vi "Initialize Hardware References.vi"(8 "error in (no error)":errorcluster, 11 "Hardware Resources in":T1={"VISA Refnum in"="", "Serial Configuration"={"Baud Rate"=460800, "Flow Control"=0}, "Voltage Level (0V)"=0.0} {"Serial Configuration"."Flow Control" items=["None", "XON/XOFF", "RTS/CTS", "XON/XOFF & RTS/CTS", "DTR/DSR", "XON/XOFF & DTR/DSR"]; "Serial Configuration"."Baud Rate" items=["9600"=9600, "19200"=19200, "38400"=38400, "57600"=57600, "115200"=115200, "230400"=230400, "460800"=460800]}) -> (0 "error out":errorcluster, 3 "Hardware Resources out":T1={"VISA Refnum in"="", "Serial Configuration"={"Baud Rate"=460800, "Flow Control"=0}, "Voltage Level (0V)"=0.0} {"Serial Configuration"."Flow Control" items=["None", "XON/XOFF", "RTS/CTS", "XON/XOFF & RTS/CTS", "DTR/DSR", "XON/XOFF & DTR/DSR"]; "Serial Configuration"."Baud Rate" items=["9600"=9600, "19200"=19200, "38400"=38400, "57600"=57600, "115200"=115200, "230400"=230400, "460800"=460800]})   [LabVIEW 2013, in "Cal Inst Acquisition.lvlib"]
doc: "Initialize the hardware references."
uses:
  Cal Inst Acquisition.lvlib
  Hardware Configuration.ctl
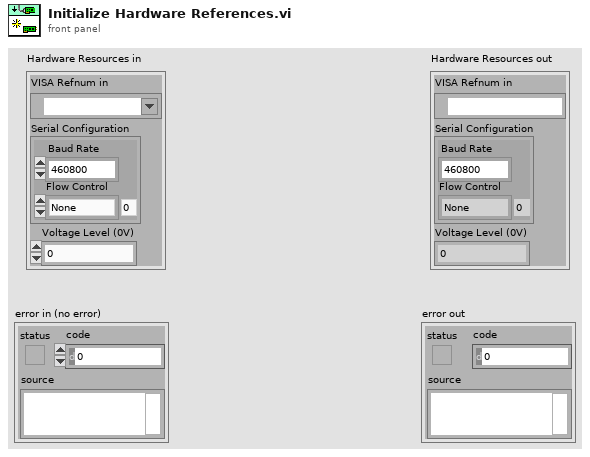
[diagram p1: front panel]
types:
  T1 = typedef "Cal Inst Acquisition.lvlib/Hardware Configuration.ctl" = cluster{"VISA Refnum in":refnum<visa-resource-name>, "Serial Configuration":cluster{"Baud Rate":u32, "Flow Control":u16}, "Voltage Level (0V)":dbl}
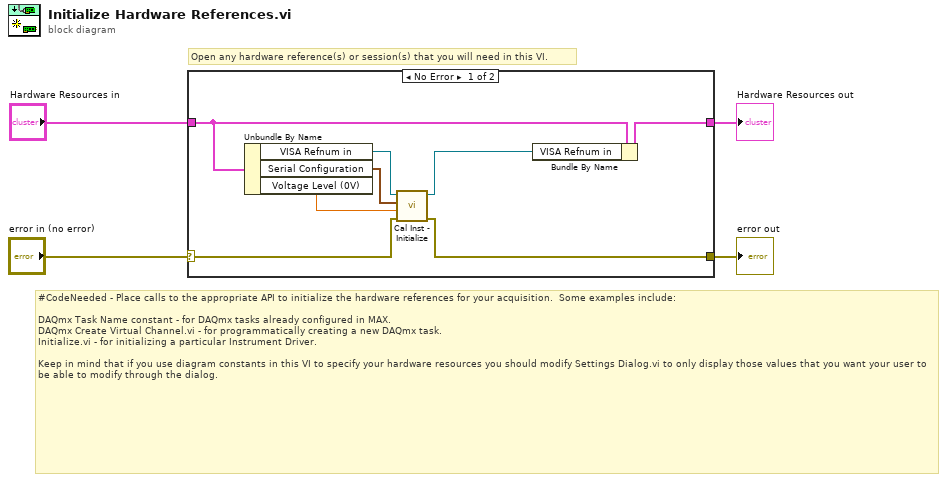
[diagram p0: block diagram]
diagram:
  # "Open any hardware reference(s) or session(s) that you will need in this VI."
  # "#CodeNeeded - Place calls to the appropriate API to initialize the hardware references for your acquisition.  Some examples include:\n\nDAQmx Task Name constant - for DAQmx tasks already configured in MAX.\nDAQmx Create Virtual Channel.vi - for programmatically creating a new DAQmx task.\nInitialize.vi - for initializing a particular Instrument Driver.\n\nKeep in mind that if you use diagram constants in this VI to specify your hardware resources you should modify Settings Dialog.vi to only display those values that you want your user to be able to modify through the dialog."
  n1 = case shown="No Error" "error in (no error)" {
    selector: "error in (no error)" -> [w6 w13]
    tunnel: [w5 w13] -> w3
    tunnel: "Hardware Resources in" -> [w11 w14]
    tunnel: [w12 w14] -> w1
    frame No Error {
      n2 = Unbundle By Name(w11) -> ("VISA Refnum in"=w8:refnum<visa-resource-name>, "Serial Configuration"=w10:cluster{"Baud Rate":u32, "Flow Control":u16}, "Voltage Level (0V)"=w9:dbl)
      n3 = call "Cal Inst - Initialize.vi"("error in (no error)"=w6, "Voltage Level (0V)"=w9, "Serial Configuration"=w10, "VISA Refnum in"=w8) -> ("error out"=w5:errorcluster, "VISA Refnum out"=w7:refnum<visa-resource-name>)  [unwired: 6 in]
      n4 = Bundle By Name(cluster=w11, "VISA Refnum in"=w7) -> (w12:T1)
    }
    frame Error {
    }
  }
  "Hardware Resources out" <- w1
  "error out" <- w3
